vi "Draw Target.vi"(1 "Cluster":T2, 2 "Color Box":u32(colorbox)=15859456, 3 "In":T1(plugin-control)) -> (0 "Out":T1(plugin-control))   [LabVIEW 2016]
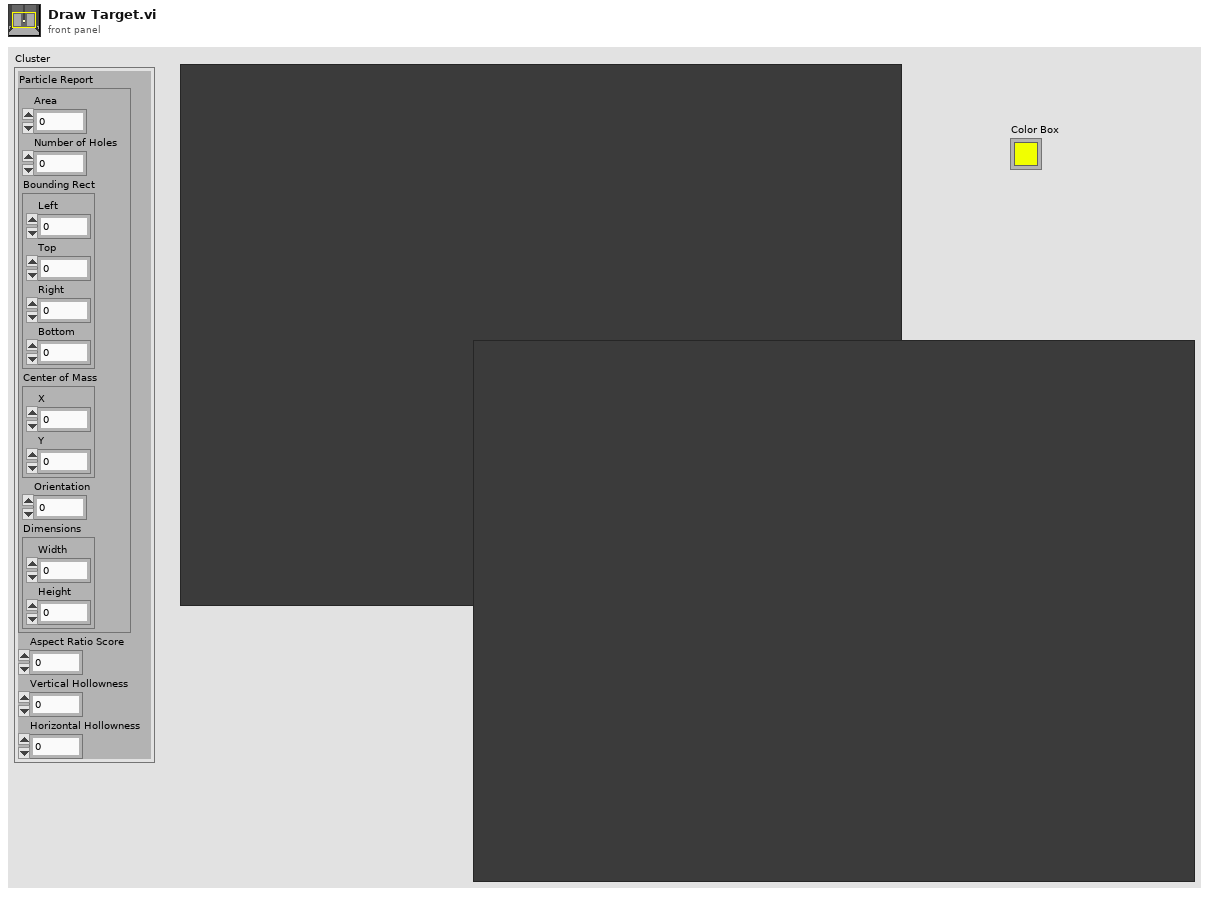
[diagram p1: front panel]
types:
  T1 = typedef "IMAQ Image.ctl" = refnum<image>
  T2 = cluster{"Particle Report":cluster{"Area":dbl, "Number of Holes":dbl, "Bounding Rect":cluster{"Left":dbl, "Top":dbl, "Right":dbl, "Bottom":dbl}, "Center of Mass":cluster{"X":dbl, "Y":dbl}, "Orientation":dbl, "Dimensions":cluster{"Width":dbl, "Height":dbl}}, "Aspect Ratio Score":dbl, "Vertical Hollowness":dbl, "Horizontal Hollowness":dbl}
  T3 = cluster{"Left":dbl, "Top":dbl, "Right":dbl, "Bottom":dbl}
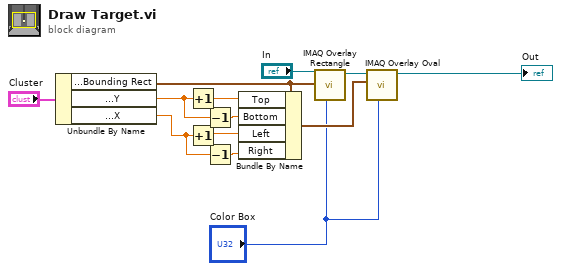
[diagram p0: block diagram]
diagram:
  n1 = Unbundle By Name("Cluster") -> ("Particle Report.Bounding Rect"=w10:T3, "Particle Report.Center of Mass.Y"=w7:dbl, "Particle Report.Center of Mass.X"=w4:dbl)
  n2 = Increment(x=w7) -> (x+1=w9:dbl)
  n3 = Increment(x=w4) -> (x+1=w5:dbl)
  n4 = Decrement(x=w7) -> (x-1=w8:dbl)
  n5 = Decrement(x=w4) -> (x-1=w6:dbl)
  n6 = Bundle By Name(cluster=w10, "Top"=w9, "Bottom"=w8, "Left"=w5, "Right"=w6) -> (w3:T3)
  n7 = call "IMAQ Overlay Rectangle"("Color"="Color Box", "Rectangle"=w10, "Image"="In") -> ("Image Out"=w11:T1)  [unwired: 7 in, 1 out]
  n8 = call "IMAQ Overlay Oval"("Color"="Color Box", "Bounding Rectangle"=w3, "Image"=w11) -> ("Image Out"=→"Out":T1)  [unwired: 7 in, 1 out]
